vi "Get Virtual DMA Address.vi"(10 "Address2":u32, 11 "Address1":u32) -> (1 "function return":u32, 2 "Address2 out":u32, 3 "Address1 out":u32)   [LabVIEW 2018, in "Copy of Andor SDK.lvlib"]
doc: "EXPNETTYPE unsigned int WINAPI GetVirtualDMAAddress(void ** Address1, void ** Address2);"
uses:
  Copy of Andor SDK.lvlib
  <userlib>/Andor SDK/ATMCD32D.dll
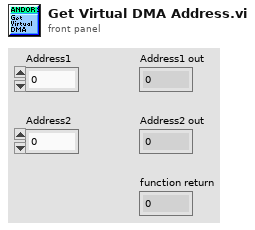
[diagram p1: front panel]
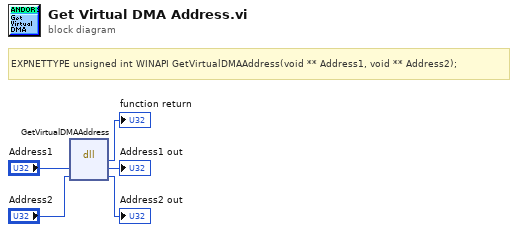
[diagram p0: block diagram]
diagram:
  # "EXPNETTYPE unsigned int WINAPI GetVirtualDMAAddress(void ** Address1, void ** Address2);"
  n1 = dll-call lib="C:/Program Files (x86)/National Instruments/LabVIEW 2018/user.lib/Andor SDK/ATMCD32D.*" fn="GetVirtualDMAAddress"("Address1"="Address1", "Address2"="Address2") -> (→"function return":u32, "Address1"=→"Address1 out":u32, "Address2"=→"Address2 out":u32)  [unwired: 3 in, 2 out]
